vi "Read Register.vi"() -> ()   [LabVIEW 2020]
uses:
  g_industrial_cam/Camera/Camera.lvclass/Camera.ctl
  g_industrial_cam/Camera/GetSetRegister.vi
  g_industrial_cam/Camera/Check Not Disconnected.vi
  <vilib>/Utility/error.llb/Error Cluster From Error Code.vi
  g_industrial_cam/Camera/Camera.lvclass
panel:
  out "Bytes Out 2":string
  out "Bytes Out":string
  out "error out":errorcluster
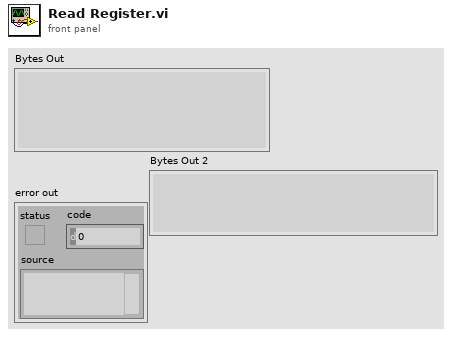
[diagram p1: front panel]
types:
  T1 = typedef "Device Enumeration.ctl" = cluster{"ID":string, "Protocol":string, "Vendor":string, "Model":string, "Serial":string, "Address":string}
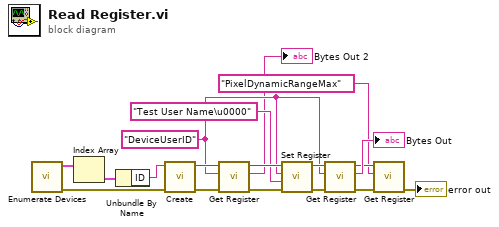
[diagram p0: block diagram]
diagram:
  w7 = "DeviceUserID" ("Register Name")
  n1 = call "Enumerate Devices.vi"() -> ("error out"=w16:errorcluster, "Devices"=w18:T1[])  [unwired: 10 in]
  n2 = Index Array(array=w18) -> (element=w17:T1)  [unwired: 1 in]
  n3 = Unbundle By Name(w17) -> ("ID"=w15:string)
  n4 = call "Create.vi"("error in (no error)"=w16, "Identifier (ID, IP etc)"=w15) -> ("error out"=w13:errorcluster, "Camera"=w14:refnum<class "Camera.lvclass">)  [unwired: 8 in]
  n5 = call "Get Register.vi"("error in (no error)"=w13, "Feature Name"=w7, "Camera in"=w14) -> ("error out"=w11:errorcluster, "Bytes Out"=→"Bytes Out 2":string, "Camera"=w12:refnum<class "Camera.lvclass">)  [unwired: 6 in]
  n6 = call "Set Register.vi"("error in (no error)"=w11, "Bytes in"="Test User Name\u0000", "Feature Name"=w7, "Camera in"=w12) -> ("error out"=w9:errorcluster, "Camera"=w8:refnum<class "Camera.lvclass">)  [unwired: 6 in]
  n7 = call "Get Register.vi"("error in (no error)"=w9, "Feature Name"=w7, "Camera in"=w8) -> ("error out"=w4:errorcluster, "Bytes Out"=→"Bytes Out":string, "Camera"=w5:refnum<class "Camera.lvclass">)  [unwired: 6 in]
  n8 = call "Get Register.vi"("error in (no error)"=w4, "Feature Name"="PixelDynamicRangeMax", "Camera in"=w5) -> ("error out"=→"error out":errorcluster)  [unwired: 6 in, 2 out]
